vi "Initialize Instrument.vi"(8 "error in (no error)":errorcluster, 10 "Reset":bool, 11 "Agilent DSO1000 in":refnum<class "Agilent DSO1000.lvclass">) -> (0 "error out":errorcluster, 3 "Agilent DSO1000 out":refnum<class "Agilent DSO1000.lvclass">)   [LabVIEW 2020, in "Agilent DSO1000.lvclass"]
uses:
  Agilent DSO1000.lvclass
  C:/Sandbox/RF Bench/Source Code/WiSpry Test Framework/Instruments/Instrument.lvclass
  Instrument.lvclass/Instrument.ctl
  <instrlib>/Agilent DSO1000 Series/Agilent DSO1000 Series.lvlib
  Instrument.lvclass
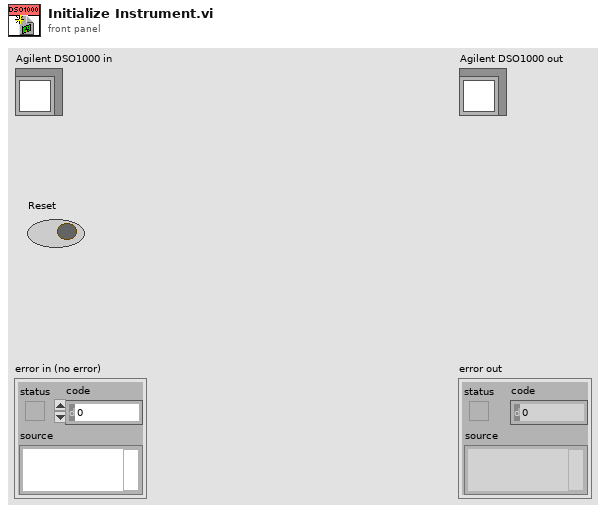
[diagram p1: front panel]
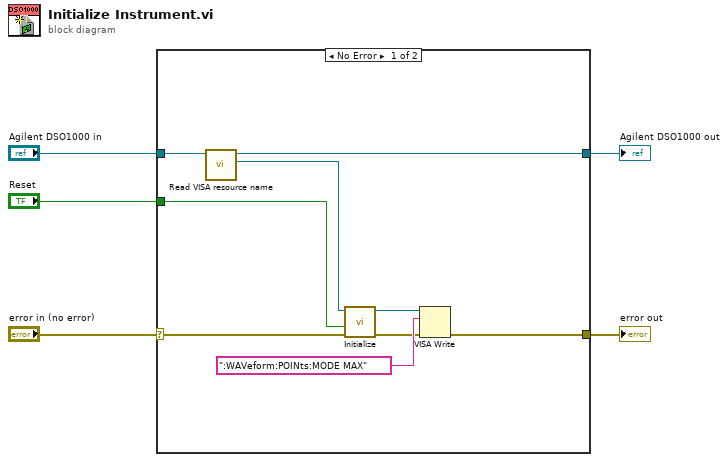
[diagram p0: block diagram]
diagram:
  n1 = case shown="No Error" "error in (no error)" {
    selector: "error in (no error)" -> [w14 w16]
    tunnel: [w7 w16] -> w4
    tunnel: [w12 w15] -> w3
    tunnel: "Agilent DSO1000 in" -> [w13 w15]
    tunnel: "Reset" -> [w10 _]
    frame No Error {
      n2 = call "Read VISA resource name.vi"("Instrument in"=w13) -> ("VISA resource name"=w11:refnum<visa-resource-name>, "Instrument out"=w12:refnum<class "Agilent DSO1000.lvclass">)  [unwired: 9 in]
      n3 = call <instrlib>:"Initialize.vi"("error in (no error)"=w14, "Reset (True)"=w10, "VISA resource name"=w11) -> ("error out"=w6:errorcluster, "VISA resource name out"=w8:refnum<visa-resource-name>)  [unwired: 7 in]
      n4 = VISA Write(VISA resource name=w8, write buffer=":WAVeform:POINts:MODE MAX", error in (no error)=w6) -> (error out=w7:errorcluster)  [unwired: 2 out]
    }
    frame Error {
    }
  }
  "error out" <- w4
  "Agilent DSO1000 out" <- w3
